vi "Get Instrument Type ID.vi"(8 "error in":errorcluster, 11 "session factory in":refnum<class "Abstract_Instrument.lvclass">) -> (0 "error out":errorcluster, 2 "instrument type id":string, 3 "session factory out":refnum<class "Abstract_Instrument.lvclass">)   [LabVIEW 2020, in "Abstract_Instrument.lvlib" / "Abstract_Instrument.lvclass"]
doc: "Returns the type ID for the instrument in the pin map file. When using third party instruments not natively supported by the pin map editor, you must create a custom instrument in the pin map file and assign it a unique instrument type ID. Return the same instrument type ID from this method to access the third party instrument from within MeasurementLink."
uses:
  Abstract_Instrument.lvclass
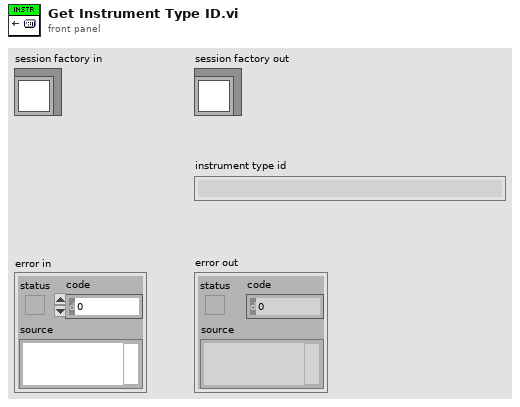
[diagram p1: front panel]
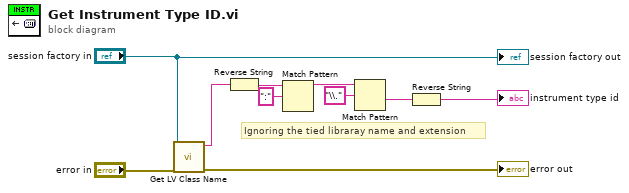
[diagram p0: block diagram]
diagram:
  # "Ignoring the tied libraray name and extension"
  n1 = call <vilib>:"Get LV Class Name.vi"("error in (no error)"="error in", "object"="session factory in") -> ("error out"=→"error out":errorcluster, "class name"=w7:string)  [unwired: 8 in]
  n2 = Reverse String(1:w7) -> (0:w6:string)
  n3 = Match Pattern(string=w6, regular expression=":") -> (before substring=w4:string)  [unwired: 1 in, 3 out]
  n4 = Match Pattern(string=w4, regular expression="\\.") -> (after substring=w2:string)  [unwired: 1 in, 3 out]
  n5 = Reverse String(1:w2) -> (0:→"instrument type id":string)
  "session factory out" <- "session factory in"
